vi "edge detect.vi"(1 "Boolean":bool) -> (0 "x .and. y?":bool)   [LabVIEW 2023]
panel:
  in  "Boolean 2":bool
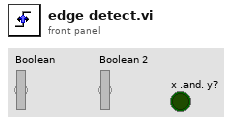
[diagram p1: front panel]
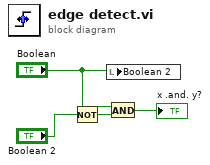
[diagram p0: block diagram]
diagram:
  n1 = Not(x="Boolean 2") -> (.not. x?=w2:bool)
  n2 = local write "Boolean 2"("Boolean") -> ()
  n3 = And(x="Boolean", y=w2) -> (x .and. y?=→"x .and. y?":bool)
